vi "Data to String (Tag Query).vi"(0 "tag path":string, 1 "data type":T2, 5 "aggregate values":T1, 7 "current value":string, 9 "time stamp":timestamp, 11 "error in (no error)":errorcluster) -> (4 "tag string array":string[](array[string]), 15 "error out":errorcluster)   [LabVIEW 2020, in "FlexLoggerTagHelpers.lvlib"]
doc: "Converts data to strings to display on the Host front panel."
uses:
  FlexLoggerTagHelpers.lvlib
  <vilib>/Skyline/Tag/Shared/typedefs/DataType.ctl
  <vilib>/Skyline/Tag/Shared/typedefs/Aggregates Double.ctl
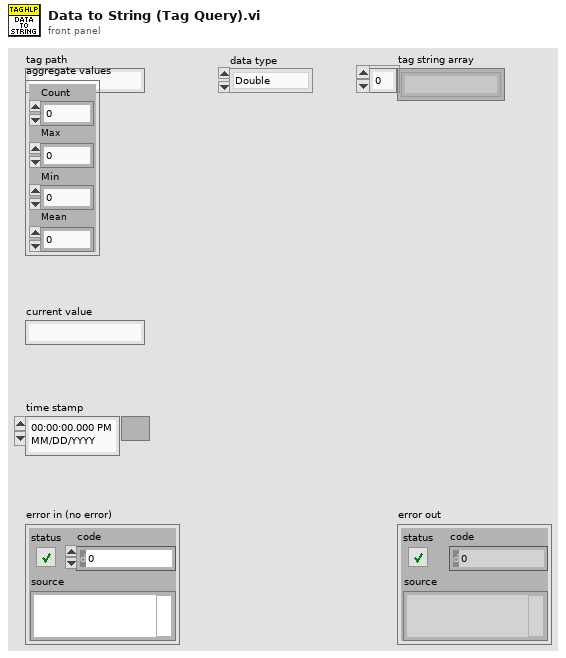
[diagram p1: front panel]
types:
  T1 = typedef "NI Skyline Tag.lvlib/Aggregates Double.ctl" = cluster{"Count":i32, "Max":dbl, "Min":dbl, "Mean":dbl}
  T2 = typedef "NI Skyline Tag.lvlib/DataType.ctl" = enum32{"Double", "I32", "String", "Boolean", "U64", "Timestamp"}
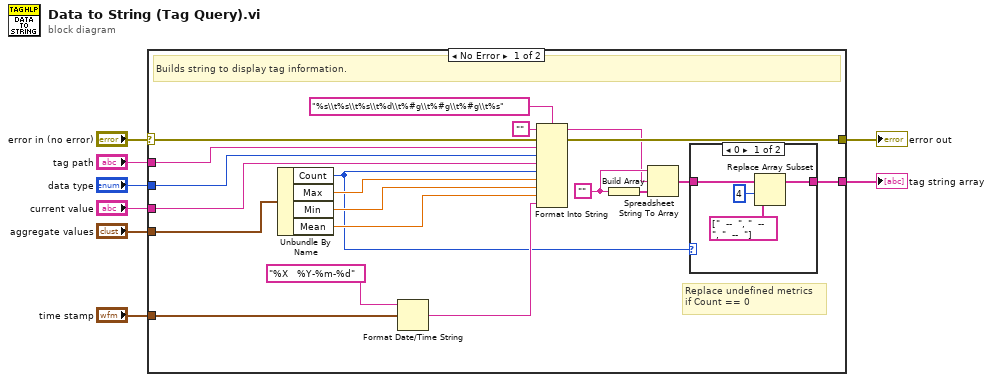
[diagram p0: block diagram]
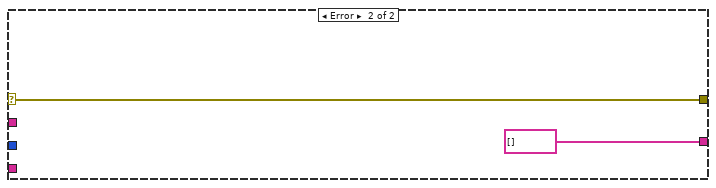
[diagram p3: hidden frame]
diagram:
  n1 = case shown="No Error" "error in (no error)" {
    selector: "error in (no error)" -> [w27 w35]
    tunnel: [w28 w35] -> w8
    tunnel: "data type" -> [w26 _]
    tunnel: "tag path" -> [w25 _]
    tunnel: "current value" -> [w24 _]
    tunnel: "aggregate values" -> [w23 _]
    tunnel: "time stamp" -> [w22 _]
    tunnel: [w9 string[] []] -> w2
    frame No Error {
      w14 = ""
      # "Replace undefined metrics\nif Count == 0"
      # "Builds string to display tag information."
      n2 = Unbundle By Name(w23) -> ("Count"=w11:i32, "Max"=w19:dbl, "Min"=w18:dbl, "Mean"=w17:dbl)
      n3 = Format Date/Time String(time format string (%c)="%X   %Y-%m-%d", seconds (now)=w22) -> (date/time string=w12:string)  [unwired: 1 in]
      n4 = Format Into String(format string="%s\\t%s\\t%s\\t%d\\t%#g\\t%#g\\t%#g\\t%s", initial string="", error in=w27, w25, w26, w24, w11, w19, w18, w17, w12) -> (resulting string=w13:string, error out=w28:errorcluster)
      n5 = Build Array(w14) -> (w15:string[])
      n6 = Spreadsheet String To Array(format string=w14, spreadsheet string=w13, array type (2D Dbl)=w15) -> (array=w10:string[])  [unwired: 1 in]
      n7 = case shown="0" w11 {
        tunnel: w10 -> [w31 w33]
        tunnel: [w29 w33] -> w9
        frame 0 {
          n8 = Replace Array Subset(array=w31, new element=string[] ["  --  ", "  --  ", "  --  "], index=4) -> (w29:string[])
        }
        frame 1, Default {
        }
      }
    }
    frame Error {
    }
  }
  "error out" <- w8
  "tag string array" <- w2
